vi "Version_4.9_8_on-chip_valves_for25ulSyringe_withModfied_Plunging.vi"() -> ()   [LabVIEW 2020] (continued)
                                n6529 = local write "Initial Plunger Position"(w6934) -> ()
                                }
                                frame #26 {
                                # "Switch to Port-10"
                                # "Port-10 of the pump is conncted to column-2 of chip"
                                n6530 = local read "VISA Refnum in\nfor Pump"() -> (w6937:refnum<visa-resource-name>)
                                n6531 = call "PortChanger (SubVI).vi"("Port Number"="10", "VISA Refnum in"=w6937) -> ()  [unwired: 10 in]
                                }
                                frame #27 {
                                n6532 = local read "Stopper that ends \nthe main loops"() -> (w6938:bool)
                                n6533 = local read "VISA Refnum in\nfor Pump"() -> (w6939:refnum<visa-resource-name>)
                                n6534 = call "ProcessCompletionWaiter (SubVI).vi"("VISA Refnum in"=w6939) -> ()  [unwired: 11 in]
                                n6535 = case shown="True" w6938 {
                                frame False {
                                }
                                frame True {
                                n6536 = local read "VISA Refnum in\nfor Pump"() -> (w6940:refnum<visa-resource-name>)
                                n6537 = call "HardStopCurrentProcess (SubVI).vi"("VISA Refnum in"=w6940) -> ()  [unwired: 11 in]
                                }
                                }
                                }
                                frame #28 {
                                # "Keeps the AMF valve after column-1 open and valve after column-2 closed"
                                n6538 = local read "Buffer-C2 Dispense\nFlow Rate (ul/min)"() -> (w6953:dbl)
                                n6539 = local read "Buffer-C2 Pumping\nResolution"() -> (w6952:T2)
                                n6540 = local read "VISA Refnum in\nfor Pump"() -> (w6955:refnum<visa-resource-name>)
                                n6541 = local write "Pause Data Collection"(FALSE ("Pause Data Collection")) -> ()
                                n6542 = local read "Volume of Syringe"() -> (w6954:dbl)
                                n6543 = call "GoToAbsolutePosition(SubVI).vi"("Absolute Volume Position in Syringe (in ul)"=0.0 ("Volume to be Dispensed"), "Volume of Syringe"=w6954, "Resolution of Pumping"=w6952, "Flow Rate (ul/min)"=w6953, "VISA Refnum in"=w6955) -> ()  [unwired: 6 in, 1 out]
                                n6544 = local read "VISA Refnum in\nfor Valve"() -> (w6949:refnum<visa-resource-name>)
                                n6545 = local read "External Valve \nOPEN"() -> (w6948:string)
                                n6546 = local write "Valve V1 Open"(FALSE ("Valve V1 Open")) -> ()
                                n6547 = local write "Valve V2 Open"(TRUE ("Valve V2 Open")) -> ()
                                n6548 = local write "Valve V3 Open"(TRUE ("Valve V3 Open")) -> ()
                                n6549 = local write "Valve V4 Open"(FALSE ("Valve V4 Open")) -> ()
                                n6550 = call "PortChanger_Valve (SubVI).vi"("Port Number"=w6948, "VISA Refnum in"=w6949) -> ()  [unwired: 10 in]
                                n6551 = local write "Valve V5 Open"(FALSE ("Valve V5 Open")) -> ()
                                n6552 = local write "Valve V6 Open"(FALSE ("Valve V6 Open")) -> ()
                                n6553 = local write "Valve V7 Open"(FALSE ("Valve V7 Open")) -> ()
                                }
                                frame #29 {
                                n6554 = local read "Initial Plunger Position"() -> (w6959:dbl)
                                n6555 = local read "Buffer-C2 Pumping\nResolution"() -> (w6958:T2)
                                n6556 = local read "VISA Refnum in\nfor Pump"() -> (w6960:refnum<visa-resource-name>)
                                n6557 = local read "Volume of Syringe"() -> (w6957:dbl)
                                n6558 = while {
                                tunnel: w6959 -> [w6966]
                                tunnel: w6960 -> [w6965]
                                tunnel: w6958 -> [w6964]
                                tunnel: w6957 -> [w6963]
                                stop <- w6961 stop-if-true
                                n6559 = Wait (ms)(milliseconds to wait=u32 100) -> ()  [unwired: 1 out]
                                n6560 = stacked-sequence {
                                tunnel: w6966 -> [w6972 _]
                                tunnel: w6965 -> [w6971 w6998]
                                tunnel: w6964 -> [w6970 _]
                                tunnel: w6963 -> [w6969 _]
                                tunnel: [_ w6994] -> w6961
                                frame #0 {
                                n6561 = call "AbsolutePlungerPosition (SubVI).vi"("VISA Refnum in"=w6971) -> ("Plunger Position"=w6968:i32)  [unwired: 10 in]
                                n6562 = case shown="\"Standard Pumping\", Default" w6970 {
                                tunnel: w6972 -> [w6977 w6986]
                                tunnel: w6968 -> [w6978 w6985]
                                tunnel: [w6976 w6983] -> w6967
                                tunnel: w6969 -> [w6975 w6984]
                                frame "Standard Pumping", Default {
                                n6563 = Subtract(x=w6977, y=w6978) -> (x-y=w6974:dbl)
                                n6564 = Absolute Value(x=w6974) -> (abs(x)=w6973:dbl)
                                n6565 = Multiply(x=w6973, y=w6975) -> (x*y=w6980:dbl)
                                n6566 = Divide(x=w6980, y=3000.0) -> (x/y=w6976:dbl)
                                }
                                frame "High Resolution Pumping" {
                                n6567 = Subtract(x=w6986, y=w6985) -> (x-y=w6982:dbl)
                                n6568 = Absolute Value(x=w6982) -> (abs(x)=w6981:dbl)
                                n6569 = Multiply(x=w6981, y=w6984) -> (x*y=w6988:dbl)
                                n6570 = Divide(x=w6988, y=24000.0) -> (x/y=w6983:dbl)
                                }
                                }
                                n6571 = local write "Volume being Injected \nin this process"(w6967) -> ()
                                }
                                frame #1 {
                                n6572 = local read "Stopper that ends \nthe main loops"() -> (w6995:bool)
                                n6573 = local read "Divert Buffer-C \ninto Column-2"() -> (w6996:bool)
                                n6574 = local read "Volume being Injected \nin this process"() -> (w6993:dbl)
                                n6575 = call "LSPOneStatus (SubVI).vi"("VISA Refnum in"=w6998) -> ("read buffer"=w7000:string)  [unwired: 10 in]
                                n6576 = call <vilib>:"Trim Whitespace.vi"("string"=w7000) -> ("trimmed string"=w6999:string)  [unwired: 1 in]
                                n6577 = Equal?(x=w6999, y="/0`\u0003") -> (x = y?=w6997:bool)
                                n6578 = Or(x=w6996, y=w6995) -> (x .or. y?=w6991:bool)
                                n6579 = Greater Or Equal?(x=w6993, y=2.0) -> (x >= y?=w6990:bool)
                                n6580 = Or(x=w6991, y=w6990) -> (x .or. y?=w6989:bool)
                                n6581 = Or(x=w6997, y=w6989) -> (x .or. y?=w6994:bool)
                                }
                                }
                                }
                                n6582 = local read "Stopper that ends \nthe main loops"() -> (w6956:bool)
                                n6583 = case shown="True" w6956 {
                                frame False {
                                }
                                frame True {
                                n6584 = local read "VISA Refnum in\nfor Pump"() -> (w7002:refnum<visa-resource-name>)
                                n6585 = call "HardStopCurrentProcess (SubVI).vi"("VISA Refnum in"=w7002) -> ()  [unwired: 11 in]
                                }
                                }
                                }
                                frame #30 {
                                # "Keeps the on-chip valves V4, V5 and V7 open"
                                # "Keeps the AMF valve after column-1 closed and valve after column-2 open"
                                n6586 = local write "Divert Buffer-C \ninto Column-2"(FALSE ("Divert Buffer-C \ninto Column-2")) -> ()
                                n6587 = local read "VISA Refnum in\nfor Pump"() -> (w7007:refnum<visa-resource-name>)
                                n6588 = local read "External Valve \nCLOSED"() -> (w7006:string)
                                n6589 = local write "Valve V3 Open"(FALSE ("Valve V3 Open")) -> ()
                                n6590 = local write "Valve V2 Open"(FALSE ("Valve V2 Open")) -> ()
                                n6591 = local write "Valve V1 Open"(FALSE ("Valve V1 Open")) -> ()
                                n6592 = local write "Valve V4 Open"(TRUE ("Valve V4 Open")) -> ()
                                n6593 = call "PortChanger_Valve (SubVI).vi"("Port Number"=w7006, "VISA Refnum in"=w7007) -> ()  [unwired: 10 in]
                                n6594 = local write "Valve V5 Open"(TRUE ("Valve V5 Open")) -> ()
                                n6595 = local write "Valve V6 Open"(FALSE ("Valve V6 Open")) -> ()
                                n6596 = local write "Valve V7 Open"(TRUE ("Valve V7 Open")) -> ()
                                }
                                frame #31 {
                                n6597 = local read "Initial Plunger Position"() -> (w7016:dbl)
                                n6598 = local read "Buffer-C2 Pumping\nResolution"() -> (w7015:T2)
                                n6599 = local read "VISA Refnum in\nfor Pump"() -> (w7017:refnum<visa-resource-name>)
                                n6600 = local read "Volume of Syringe"() -> (w7014:dbl)
                                n6601 = while {
                                tunnel: w7016 -> [w7023]
                                tunnel: w7017 -> [w7022]
                                tunnel: w7015 -> [w7021]
                                tunnel: w7014 -> [w7020]
                                stop <- w7018 stop-if-true
                                n6602 = Wait (ms)(milliseconds to wait=u32 100) -> ()  [unwired: 1 out]
                                n6603 = stacked-sequence {
                                tunnel: w7023 -> [w7029 _]
                                tunnel: w7022 -> [w7028 w7051]
                                tunnel: w7021 -> [w7027 _]
                                tunnel: w7020 -> [w7026 _]
                                tunnel: [_ w7049] -> w7018
                                frame #0 {
                                n6604 = call "AbsolutePlungerPosition (SubVI).vi"("VISA Refnum in"=w7028) -> ("Plunger Position"=w7025:i32)  [unwired: 10 in]
                                n6605 = case shown="\"Standard Pumping\", Default" w7027 {
                                tunnel: w7029 -> [w7034 w7043]
                                tunnel: w7025 -> [w7035 w7042]
                                tunnel: [w7033 w7040] -> w7024
                                tunnel: w7026 -> [w7032 w7041]
                                frame "Standard Pumping", Default {
                                n6606 = Subtract(x=w7034, y=w7035) -> (x-y=w7031:dbl)
                                n6607 = Absolute Value(x=w7031) -> (abs(x)=w7030:dbl)
                                n6608 = Multiply(x=w7030, y=w7032) -> (x*y=w7037:dbl)
                                n6609 = Divide(x=w7037, y=3000.0) -> (x/y=w7033:dbl)
                                }
                                frame "High Resolution Pumping" {
                                n6610 = Subtract(x=w7043, y=w7042) -> (x-y=w7039:dbl)
                                n6611 = Absolute Value(x=w7039) -> (abs(x)=w7038:dbl)
                                n6612 = Multiply(x=w7038, y=w7041) -> (x*y=w7045:dbl)
                                n6613 = Divide(x=w7045, y=24000.0) -> (x/y=w7040:dbl)
                                }
                                }
                                n6614 = local write "Volume being Injected \nin this process"(w7024) -> ()
                                }
                                frame #1 {
                                n6615 = call "LSPOneStatus (SubVI).vi"("VISA Refnum in"=w7051) -> ("read buffer"=w7053:string)  [unwired: 10 in]
                                n6616 = call <vilib>:"Trim Whitespace.vi"("string"=w7053) -> ("trimmed string"=w7052:string)  [unwired: 1 in]
                                n6617 = Equal?(x=w7052, y="/0`\u0003") -> (x = y?=w7050:bool)
                                n6618 = local read "Stopper that ends \nthe main loops"() -> (w7047:bool)
                                n6619 = local read "Divert Sample \nonto Grid"() -> (w7048:bool)
                                n6620 = Or(x=w7048, y=w7047) -> (x .or. y?=w7046:bool)
                                n6621 = Or(x=w7050, y=w7046) -> (x .or. y?=w7049:bool)
                                }
                                }
                                }
                                n6622 = local read "Stopper that ends \nthe main loops"() -> (w7013:bool)
                                n6623 = case shown="True" w7013 {
                                frame False {
                                }
                                frame True {
                                n6624 = local read "VISA Refnum in\nfor Pump"() -> (w7055:refnum<visa-resource-name>)
                                n6625 = call "HardStopCurrentProcess (SubVI).vi"("VISA Refnum in"=w7055) -> ()  [unwired: 11 in]
                                }
                                }
                                }
                                frame #32 {
                                n6626 = local read "Volume being Injected \nin this process"() -> (w7058:dbl)
                                n6627 = local read "VISA Refnum in\nfor Pump"() -> (w7060:refnum<visa-resource-name>)
                                n6628 = call "AbsolutePlungerPosition (SubVI).vi"("VISA Refnum in"=w7060) -> ("Plunger Position"=w7059:i32)  [unwired: 10 in]
                                n6629 = local write "Pause Data Collection"(TRUE) -> ()
                                n6630 = local write "True Volume being \ninjected in this\nprocess"(w7058) -> ()
                                n6631 = local write "Position\nNow"(w7059) -> ()
                                n6632 = Wait (ms)(milliseconds to wait=u32 500) -> ()  [unwired: 1 out]
                                }
                                frame #33 {
                                # "Sample Deposition onto EM-Grid"
                                n6633 = local read "Divert Sample \nonto Grid"() -> (w7061:bool)
                                n6634 = case shown="True" w7061 {
                                frame False {
                                }
                                frame True {
                                n6635 = stacked-sequence {
                                frame #0 {
                                # "Discard the initial volume of fluid that is present in the channel prior to detection"
                                n6636 = local read "Buffer-C2 Pumping\nResolution"() -> (w7072:T2)
                                n6637 = local read "Initial Plunger Position"() -> (w7071:dbl)
                                n6638 = local read "VISA Refnum in\nfor Pump"() -> (w7073:refnum<visa-resource-name>)
                                n6639 = local read "Position\nNow"() -> (w7069:dbl)
                                n6640 = local read "Volume of Syringe"() -> (w7070:dbl)
                                n6641 = local write "Pause Data Collection"(FALSE) -> ()
                                n6642 = while {
                                tunnel: w7073 -> [w7083]
                                tunnel: w7072 -> [w7082]
                                tunnel: w7071 -> [w7078]
                                tunnel: w7070 -> [w7081]
                                tunnel: w7069 -> [w7077]
                                stop <- w7079 stop-if-true
                                n6643 = stacked-sequence {
                                tunnel: w7083 -> [w7089 w7111 w7143]
                                tunnel: w7082 -> [w7088 w7110 _]
                                tunnel: w7078 -> [w7086 _ _]
                                tunnel: w7081 -> [w7085 w7108 _]
                                tunnel: [_ _ w7137] -> w7079
                                tunnel: w7077 -> [_ w7106 _]
                                frame #0 {
                                # "From here on 'True Volume being injected \nin this process' represents the true total \nvolume in this process"
                                n6644 = call "AbsolutePlungerPosition (SubVI).vi"("VISA Refnum in"=w7089) -> ("Plunger Position"=w7087:i32)  [unwired: 10 in]
                                n6645 = case shown="..\"Standard Pumping\"" w7088 {
                                tunnel: w7087 -> [w7097 w7105]
                                tunnel: w7086 -> [w7096 w7104]
                                tunnel: w7085 -> [w7093 w7101]
                                tunnel: [w7090 w7098] -> w7084
                                frame .."Standard Pumping" {
                                n6646 = Subtract(x=w7097, y=w7096) -> (x-y=w7095:dbl)
                                n6647 = Absolute Value(x=w7095) -> (abs(x)=w7094:dbl)
                                n6648 = Multiply(x=w7094, y=w7093) -> (x*y=w7092:dbl)
                                n6649 = Divide(x=w7092, y=3000.0) -> (x/y=w7090:dbl)
                                }
                                frame "High Resolution Pumping".. {
                                n6650 = Subtract(x=w7105, y=w7104) -> (x-y=w7103:dbl)
                                n6651 = Absolute Value(x=w7103) -> (abs(x)=w7102:dbl)
                                n6652 = Multiply(x=w7102, y=w7101) -> (x*y=w7100:dbl)
                                n6653 = Divide(x=w7100, y=24000.0) -> (x/y=w7098:dbl)
                                }
                                }
                                n6654 = local write "True Volume being \ninjected in this\nprocess"(w7084) -> ()
                                }
                                frame #1 {
                                # "From here on 'Volume being injected \nin this process' represents the volume \nin this sub process"
                                n6655 = call "AbsolutePlungerPosition (SubVI).vi"("VISA Refnum in"=w7111) -> ("Plunger Position"=w7109:i32)  [unwired: 10 in]
                                n6656 = case shown="..\"Standard Pumping\"" w7110 {
                                tunnel: w7109 -> [w7119 w7127]
                                tunnel: w7106 -> [w7118 w7126]
                                tunnel: w7108 -> [w7115 w7123]
                                tunnel: [w7112 w7120] -> w7107
                                frame .."Standard Pumping" {
                                n6657 = Subtract(x=w7119, y=w7118) -> (x-y=w7117:dbl)
                                n6658 = Absolute Value(x=w7117) -> (abs(x)=w7116:dbl)
                                n6659 = Multiply(x=w7116, y=w7115) -> (x*y=w7114:dbl)
                                n6660 = Divide(x=w7114, y=3000.0) -> (x/y=w7112:dbl)
                                }
                                frame "High Resolution Pumping".. {
                                n6661 = Subtract(x=w7127, y=w7126) -> (x-y=w7125:dbl)
                                n6662 = Absolute Value(x=w7125) -> (abs(x)=w7124:dbl)
                                n6663 = Multiply(x=w7124, y=w7123) -> (x*y=w7122:dbl)
                                n6664 = Divide(x=w7122, y=24000.0) -> (x/y=w7120:dbl)
                                }
                                }
                                n6665 = local write "Volume being Injected \nin this process"(w7107) -> ()
                                }
                                frame #2 {
                                n6666 = local read "Discard Volume"() -> (w7131:dbl)
                                n6667 = local read "Discard fluid \nprior to 1st \ndeposition"() -> (w7136:bool)
                                n6668 = local read "Volume being Injected \nin this process"() -> (w7135:dbl)
                                n6669 = Greater Or Equal?(x=w7135, y=w7131) -> (x >= y?=w7133:bool)
                                n6670 = call "AbsolutePlungerPositionStatus (SubVI).vi"("VISA Refnum in"=w7143) -> ("read buffer"=w7142:string)  [unwired: 10 in]
                                n6671 = local read "Stop for End of \nExperiment \nand Data Writing"() -> (w7129:bool)
                                n6672 = call <vilib>:"Trim Whitespace.vi"("string"=w7142) -> ("trimmed string"=w7141:string)  [unwired: 1 in]
                                n6673 = Not(x=w7136) -> (.not. x?=w7134:bool)
                                n6674 = Equal?(x=w7141, y="/0`\u0003") -> (x = y?=w7139:bool)
                                n6675 = Or(x=w7134, y=w7133) -> (x .or. y?=w7132:bool)
                                n6676 = local read "Re-SEC"() -> (w7130:bool)
                                n6677 = Or(x=w7129, y=w7130) -> (x .or. y?=w7128:bool)
                                n6678 = Or(x=w7132, y=w7128) -> (x .or. y?=w7138:bool)
                                n6679 = Or(x=w7139, y=w7138) -> (x .or. y?=w7137:bool)
                                }
                                }
                                n6680 = Wait (ms)(milliseconds to wait=u32 100) -> ()  [unwired: 1 out]
                                }
                                n6681 = local write "Valve V4 Open"(TRUE ("Valve V4 Open")) -> ()
                                n6682 = local write "Valve V3 Open"(FALSE ("Valve V3 Open")) -> ()
                                n6683 = local write "Valve V2 Open"(FALSE ("Valve V2 Open")) -> ()
                                n6684 = local write "Valve V1 Open"(FALSE ("Valve V1 Open")) -> ()
                                n6685 = local write "Valve V5 Open"(TRUE ("Valve V5 Open")) -> ()
                                n6686 = local write "Valve V6 Open"(TRUE ("Valve V6 Open")) -> ()
                                n6687 = local write "Valve V7 Open"(FALSE ("Valve V7 Open")) -> ()
                                n6688 = local write "Volume being Injected \nin this process"(0.0) -> ()
                                }
                                frame #1 {
                                # "Keeps the on-chip valve V1, V2 and V3 closed,\nHalts also deposition onto the grid\nand waits for the 1st redeposit command. Once the command is issued\nit starts pumpoing and moves onto the next frame"
                                n6689 = stacked-sequence {
                                frame #0 {
                                n6690 = local write "Valve V5 Open"(FALSE ("Valve V5 Open")) -> ()
                                n6691 = local write "Valve V1 Open"(FALSE ("Valve V1 Open")) -> ()
                                n6692 = local read "VISA Refnum in\nfor Pump"() -> (w7153:refnum<visa-resource-name>)
                                n6693 = local write "Valve V2 Open"(FALSE ("Valve V2 Open")) -> ()
                                n6694 = local write "Valve V6 Open"(FALSE ("Valve V6 Open")) -> ()
                                n6695 = local write "Re-deposit Sample\nonto Grid"(FALSE ("Redeposit Sample\nonto Grid")) -> ()
                                n6696 = local write "Pause Data Collection"(TRUE ("Pause Data Collection")) -> ()
                                n6697 = call "HardStopCurrentProcess (SubVI).vi"("VISA Refnum in"=w7153) -> ()  [unwired: 11 in]
                                n6698 = local write "Valve V7 Open"(FALSE ("Valve V7 Open")) -> ()
                                n6699 = local write "Valve V3 Open"(FALSE ("Valve V3 Open")) -> ()
                                n6700 = local write "Valve V4 Open"(FALSE ("Valve V4 Open")) -> ()
                                }
                                frame #1 {
                                n6701 = while {
                                stop <- w7159 stop-if-true
                                n6702 = local read "Stop for End of \nExperiment \nand Data Writing"() -> (w7157:bool)
                                n6703 = local read "Re-deposit Sample\nonto Grid"() -> (w7160:bool)
                                n6704 = local read "Re-SEC"() -> (w7158:bool)
                                n6705 = Or(x=w7157, y=w7158) -> (x .or. y?=w7156:bool)
                                n6706 = Or(x=w7160, y=w7156) -> (x .or. y?=w7159:bool)
                                }
                                n6707 = local write "Discard fluid \nprior to 1st \ndeposition"(FALSE ("Discard fluid \nprior to 1st \ndeposition")) -> ()
                                n6708 = One Button Dialog(message="Do you want to deposit sample on another grid? If yes, turn on 'Re-deposit Sample onto Grid'. Else turn on Re-SEC to do SEC again or STOP to end the experiment") -> ()  [unwired: 1 in, 1 out]
                                }
                                frame #2 {
                                n6709 = local write "Valve V6 Open"(TRUE ("Valve V3 Open")) -> ()
                                n6710 = local write "Valve V4 Open"(TRUE ("Valve V1 Open")) -> ()
                                n6711 = local write "Valve V5 Open"(TRUE ("Valve V2 Open")) -> ()
                                n6712 = local write "Valve V7 Open"(FALSE ("Valve V7 Open")) -> ()
                                }
                                frame #3 {
                                n6713 = local read "Re-deposit Sample\nonto Grid"() -> (w7165:bool)
                                n6714 = case shown="True" w7165 {
                                frame False {
                                n6715 = local write "Suction On/Off"(FALSE ("Suction On/Off")) -> ()
                                }
                                frame True {
                                n6716 = stacked-sequence {
                                frame #0 {
                                n6717 = local read "VISA Refnum in\nfor Pump"() -> (w7168:refnum<visa-resource-name>)
                                n6718 = call "AbsolutePlungerPosition (SubVI).vi"("VISA Refnum in"=w7168) -> ("Plunger Position"=w7167:i32)  [unwired: 10 in]
                                n6719 = local write "Position\nNow"(w7167) -> ()
                                }
                                frame #1 {
                                n6720 = local read "Buffer-C2 Pumping\nResolution"() -> (w7170:T2)
                                n6721 = case shown="\"Standard Pumping\", Default" w7170 {
                                tunnel: [w7171 w7182] -> w7169
                                frame "Standard Pumping", Default {
                                n6722 = local read "Buffer-C2 Volume \nto be Pumped"() -> (w7174:dbl)
                                n6723 = local read "Volume of Syringe"() -> (w7177:dbl)
                                n6724 = local read "Initial Plunger Position"() -> (w7181:dbl)
                                n6725 = local read "Position\nNow"() -> (w7180:dbl)
                                n6726 = Subtract(x=w7181, y=w7180) -> (x-y=w7179:dbl)
                                n6727 = Absolute Value(x=w7179) -> (abs(x)=w7178:dbl)
                                n6728 = Multiply(x=w7178, y=w7177) -> (x*y=w7176:dbl)
                                n6729 = Divide(x=w7176, y=3000.0) -> (x/y=w7173:dbl)
                                n6730 = Subtract(x=w7173, y=w7174) -> (x-y=w7172:dbl)
                                n6731 = Absolute Value(x=w7172) -> (abs(x)=w7171:dbl)
                                }
                                frame "High Resolution Pumping" {
                                n6732 = local read "Buffer-C2 Volume \nto be Pumped"() -> (w7185:dbl)
                                n6733 = local read "Volume of Syringe"() -> (w7188:dbl)
                                n6734 = local read "Initial Plunger Position"() -> (w7192:dbl)
                                n6735 = local read "Position\nNow"() -> (w7191:dbl)
                                n6736 = Subtract(x=w7192, y=w7191) -> (x-y=w7190:dbl)
                                n6737 = Absolute Value(x=w7190) -> (abs(x)=w7189:dbl)
                                n6738 = Multiply(x=w7189, y=w7188) -> (x*y=w7187:dbl)
                                n6739 = Divide(x=w7187, y=24000.0) -> (x/y=w7184:dbl)
                                n6740 = Subtract(x=w7184, y=w7185) -> (x-y=w7183:dbl)
                                n6741 = Absolute Value(x=w7183) -> (abs(x)=w7182:dbl)
                                }
                                }
                                n6742 = local write "Buffer-C Volume\nleft to be Pumped"(w7169) -> ()
                                }
                                frame #2 {
                                n6743 = local read "Buffer-C2 Dispense\nFlow Rate (ul/min)"() -> (w7196:dbl)
                                n6744 = local read "Buffer-C2 Pumping\nResolution"() -> (w7195:T2)
                                n6745 = local read "VISA Refnum in\nfor Pump"() -> (w7198:refnum<visa-resource-name>)
                                n6746 = local read "Volume of Syringe"() -> (w7197:dbl)
                                n6747 = call "GoToAbsolutePosition(SubVI).vi"("Absolute Volume Position in Syringe (in ul)"=0.0, "Volume of Syringe"=w7197, "Resolution of Pumping"=w7195, "Flow Rate (ul/min)"=w7196, "VISA Refnum in"=w7198) -> ()  [unwired: 6 in, 1 out]
                                n6748 = local write "Suction On/Off"(FALSE ("Suction On/Off")) -> ()
                                }
                                }
                                }
                                }
                                }
                                frame #4 {
                                n6749 = local read "Stop for End of \nExperiment \nand Data Writing"() -> (w7200:bool)
                                n6750 = local read "Re-SEC"() -> (w7201:bool)
                                n6751 = Or(x=w7200, y=w7201) -> (x .or. y?=w7199:bool)
                                n6752 = case shown="True" w7199 {
                                frame False {
                                }
                                frame True {
                                n6753 = local read "VISA Refnum in\nfor Pump"() -> (w7202:refnum<visa-resource-name>)
                                n6754 = call "HardStopCurrentProcess (SubVI).vi"("VISA Refnum in"=w7202) -> ()  [unwired: 11 in]
                                }
                                }
                                }
                                }
                                }
                                frame #2 {
                                # "Keeps the on-chip valve V1, V2 Open and V3 closed"
                                n6755 = while {
                                stop <- w7208 stop-if-true
                                n6756 = local read "Suction On/Off"() -> (w7209:bool)
                                n6757 = case shown="True" w7209 {
                                frame False {
                                n6758 = local read "Buffer-C2 Pumping\nResolution"() -> (w7215:T2)
                                n6759 = local read "Initial Plunger Position"() -> (w7214:dbl)
                                n6760 = local read "VISA Refnum in\nfor Pump"() -> (w7216:refnum<visa-resource-name>)
                                n6761 = local read "Position\nNow"() -> (w7212:dbl)
                                n6762 = local read "Volume of Syringe"() -> (w7213:dbl)
                                n6763 = local write "Volume being Injected \nin this process"(0.0) -> ()
                                n6764 = local write "Pause Data Collection"(FALSE) -> ()
                                n6765 = while {
                                tunnel: w7216 -> [w7223]
                                tunnel: w7215 -> [w7222]
                                tunnel: w7214 -> [w7218]
                                tunnel: w7213 -> [w7221]
                                tunnel: w7212 -> [w7217]
                                stop <- w7219 stop-if-true
                                n6766 = stacked-sequence {
                                tunnel: w7223 -> [w7229 w7251 w7276]
                                tunnel: w7222 -> [w7228 w7250 _]
                                tunnel: w7218 -> [w7226 _ _]
                                tunnel: w7221 -> [w7225 w7248 _]
                                tunnel: [_ _ w7268] -> w7219
                                tunnel: w7217 -> [_ w7246 _]
                                frame #0 {
                                # "From here on 'True Volume being injected \nin this process' represents the true total \nvolume in this process"
                                n6767 = call "AbsolutePlungerPosition (SubVI).vi"("VISA Refnum in"=w7229) -> ("Plunger Position"=w7227:i32)  [unwired: 10 in]
                                n6768 = case shown="..\"Standard Pumping\"" w7228 {
                                tunnel: w7227 -> [w7237 w7245]
                                tunnel: w7226 -> [w7236 w7244]
                                tunnel: w7225 -> [w7233 w7241]
                                tunnel: [w7230 w7238] -> w7224
                                frame .."Standard Pumping" {
                                n6769 = Subtract(x=w7237, y=w7236) -> (x-y=w7235:dbl)
                                n6770 = Absolute Value(x=w7235) -> (abs(x)=w7234:dbl)
                                n6771 = Multiply(x=w7234, y=w7233) -> (x*y=w7232:dbl)
                                n6772 = Divide(x=w7232, y=3000.0) -> (x/y=w7230:dbl)
                                }
                                frame "High Resolution Pumping".. {
                                n6773 = Subtract(x=w7245, y=w7244) -> (x-y=w7243:dbl)
                                n6774 = Absolute Value(x=w7243) -> (abs(x)=w7242:dbl)
                                n6775 = Multiply(x=w7242, y=w7241) -> (x*y=w7240:dbl)
                                n6776 = Divide(x=w7240, y=24000.0) -> (x/y=w7238:dbl)
                                }
                                }
                                n6777 = local write "True Volume being \ninjected in this\nprocess"(w7224) -> ()
                                }
                                frame #1 {
                                # "From here on 'Volume being injected \nin this process' represents the volume \nin this sub process"
                                n6778 = call "AbsolutePlungerPosition (SubVI).vi"("VISA Refnum in"=w7251) -> ("Plunger Position"=w7249:i32)  [unwired: 10 in]
                                n6779 = case shown="..\"Standard Pumping\"" w7250 {
                                tunnel: w7249 -> [w7259 w7267]
                                tunnel: w7246 -> [w7258 w7266]
                                tunnel: w7248 -> [w7255 w7263]
                                tunnel: [w7252 w7260] -> w7247
                                frame .."Standard Pumping" {
                                n6780 = Subtract(x=w7259, y=w7258) -> (x-y=w7257:dbl)
                                n6781 = Absolute Value(x=w7257) -> (abs(x)=w7256:dbl)
                                n6782 = Multiply(x=w7256, y=w7255) -> (x*y=w7254:dbl)
                                n6783 = Divide(x=w7254, y=3000.0) -> (x/y=w7252:dbl)
                                }
                                frame "High Resolution Pumping".. {
                                n6784 = Subtract(x=w7267, y=w7266) -> (x-y=w7265:dbl)
                                n6785 = Absolute Value(x=w7265) -> (abs(x)=w7264:dbl)
                                n6786 = Multiply(x=w7264, y=w7263) -> (x*y=w7262:dbl)
                                n6787 = Divide(x=w7262, y=24000.0) -> (x/y=w7260:dbl)
                                }
                                }
                                n6788 = local write "Volume being Injected \nin this process"(w7247) -> ()
                                }
                                frame #2 {
                                n6789 = local read "Stop for End of \nExperiment \nand Data Writing"() -> (w7271:bool)
                                n6790 = local read "Suction On/Off"() -> (w7272:bool)
                                n6791 = call "AbsolutePlungerPositionStatus (SubVI).vi"("VISA Refnum in"=w7276) -> ("read buffer"=w7275:string)  [unwired: 10 in]
                                n6792 = call <vilib>:"Trim Whitespace.vi"("string"=w7275) -> ("trimmed string"=w7274:string)  [unwired: 1 in]
                                n6793 = Equal?(x=w7274, y="/0`\u0003") -> (x = y?=w7270:bool)
                                n6794 = Or(x=w7272, y=w7271) -> (x .or. y?=w7269:bool)
                                n6795 = Or(x=w7270, y=w7269) -> (x .or. y?=w7268:bool)
                                }
                                }
                                n6796 = Wait (ms)(milliseconds to wait=u32 100) -> ()  [unwired: 1 out]
                                }
                                }
                                frame True {
                                n6797 = stacked-sequence {
                                frame #0 {
                                n6798 = local read "Suction Pressure\nfor EM-grid \nDeposition (mbar)"() -> (w7281:sgl)
                                n6799 = local write "Valve V4 Open"(FALSE ("Valve V4 Open")) -> ()
                                n6800 = local read "VISA Refnum in\nfor Pump"() -> (w7284:refnum<visa-resource-name>)
                                n6801 = local write "Valve V5 Open"(FALSE ("Valve V1 Open")) -> ()
                                n6802 = local write "Suction pressure \nfor grid deposition"(w7281) -> ()
                                n6803 = local write "Re-deposit Sample\nonto Grid"(FALSE ("Redeposit Sample\nonto Grid")) -> ()
                                n6804 = local write "Pause Data Collection"(TRUE ("Pause Data Collection")) -> ()
                                n6805 = call "HardStopCurrentProcess (SubVI).vi"("VISA Refnum in"=w7284) -> ()  [unwired: 11 in]
                                n6806 = local write "Valve V6 Open"(TRUE ("Valve V2 Open")) -> ()
                                n6807 = local write "Valve V7 Open"(TRUE ("Valve V3 Open")) -> ()
                                }
                                frame #1 {
                                n6808 = call <vilib>:"fgt init.vi"() -> ("error out"=w7285:errorcluster)  [unwired: 11 in]
                                n6809 = while {
                                tunnel: [w7288] -> w7286
                                tunnel: w7285 -> [w7287]
                                stop <- w7291 stop-if-true
                                # "'5' corresponds to 2nd positin in the line-up series"
                                n6810 = local read "Stop for End of \nExperiment \nand Data Writing"() -> (w7292:bool)
                                n6811 = local read "Suction Pressure\nfor EM-grid \nDeposition (mbar)"() -> (w7289:sgl)
                                n6812 = call <vilib>:"fgt set pressure.vi"("error in (no error)"=w7287, "pressure"=w7289, "pressureIndex"=u32 1) -> ("error out"=w7288:errorcluster)  [unwired: 8 in]
                                n6813 = local read "Suction On/Off"() -> (w7294:bool)
                                n6814 = Not(x=w7294) -> (.not. x?=w7293:bool)
                                n6815 = Wait (ms)(milliseconds to wait=u32 10) -> ()  [unwired: 1 out]
                                n6816 = Or(x=w7293, y=w7292) -> (x .or. y?=w7291:bool)
                                }
                                n6817 = call <vilib>:"fgt close.vi"("error in (no error)"=w7286) -> ()  [unwired: 10 in, 1 out]
                                }
                                frame #2 {
                                n6818 = call <vilib>:"fgt init.vi"() -> ("error out"=w7297:errorcluster)  [unwired: 11 in]
                                n6819 = while {
                                tunnel: w7297 -> [w7300]
                                tunnel: [w7298] -> w7296
                                stop <- w7306 stop-if-true
                                n6820 = local read "Stop for End of \nExperiment \nand Data Writing"() -> (w7302:bool)
                                n6821 = local read "Suction On/Off"() -> (w7304:bool)
                                n6822 = call <vilib>:"fgt set pressure.vi"("error in (no error)"=w7300, "pressure"=sgl 0.0, "pressureIndex"=u32 1) -> ("error out"=w7298:errorcluster)  [unwired: 8 in]
                                n6823 = Not(x=w7304) -> (.not. x?=w7303:bool)
                                n6824 = Wait (ms)(milliseconds to wait=u32 10) -> ()  [unwired: 1 out]
                                n6825 = Or(x=w7303, y=w7302) -> (x .or. y?=w7306:bool)
                                }
                                n6826 = call <vilib>:"fgt close.vi"("error in (no error)"=w7296) -> ()  [unwired: 10 in, 1 out]
                                }
                                frame #3 {
                                n6827 = local write "Valve V7 Open"(FALSE ("Valve V3 Open")) -> ()
                                n6828 = local write "Valve V5 Open"(FALSE ("Valve V1 Open")) -> ()
                                n6829 = local write "Valve V6 Open"(FALSE ("Valve V2 Open")) -> ()
                                n6830 = local write "Valve V4 Open"(FALSE ("Valve V4 Open")) -> ()
                                }
                                frame #4 {
                                n6831 = while {
                                stop <- w7315 stop-if-true
                                n6832 = local read "Stop for End of \nExperiment \nand Data Writing"() -> (w7313:bool)
                                n6833 = local read "Re-deposit Sample\nonto Grid"() -> (w7316:bool)
                                n6834 = local read "Re-SEC"() -> (w7314:bool)
                                n6835 = Or(x=w7313, y=w7314) -> (x .or. y?=w7312:bool)
                                n6836 = Or(x=w7316, y=w7312) -> (x .or. y?=w7315:bool)
                                }
                                n6837 = One Button Dialog(message="Do you want to deposit sample on another grid? If yes, turn on 'Re-deposit Sample onto Grid'. Else turn on Re-SEC to do SEC again or STOP to end the experiment") -> ()  [unwired: 1 in, 1 out]
                                }
                                frame #5 {
                                n6838 = local write "Valve V4 Open"(TRUE ("Valve V4 Open")) -> ()
                                n6839 = local write "Valve V7 Open"(FALSE ("Valve V3 Open")) -> ()
                                n6840 = local write "Valve V5 Open"(TRUE ("Valve V1 Open")) -> ()
                                n6841 = local write "Valve V6 Open"(TRUE ("Valve V2 Open")) -> ()
                                }
                                frame #6 {
                                n6842 = local read "Re-deposit Sample\nonto Grid"() -> (w7321:bool)
                                n6843 = case shown="True" w7321 {
                                frame False {
                                n6844 = local write "Suction On/Off"(FALSE ("Suction On/Off")) -> ()
                                }
                                frame True {
                                n6845 = stacked-sequence {
                                frame #0 {
                                n6846 = local read "VISA Refnum in\nfor Pump"() -> (w7324:refnum<visa-resource-name>)
                                n6847 = call "AbsolutePlungerPosition (SubVI).vi"("VISA Refnum in"=w7324) -> ("Plunger Position"=w7323:i32)  [unwired: 10 in]
                                n6848 = local write "Position\nNow"(w7323) -> ()
                                }
                                frame #1 {
                                n6849 = local read "Buffer-C2 Pumping\nResolution"() -> (w7326:T2)
                                n6850 = case shown="\"Standard Pumping\", Default" w7326 {
                                tunnel: [w7327 w7338] -> w7325
                                frame "Standard Pumping", Default {
                                n6851 = local read "Buffer-C2 Volume \nto be Pumped"() -> (w7330:dbl)
                                n6852 = local read "Volume of Syringe"() -> (w7333:dbl)
                                n6853 = local read "Initial Plunger Position"() -> (w7337:dbl)
                                n6854 = local read "Position\nNow"() -> (w7336:dbl)
                                n6855 = Subtract(x=w7337, y=w7336) -> (x-y=w7335:dbl)
                                n6856 = Absolute Value(x=w7335) -> (abs(x)=w7334:dbl)
                                n6857 = Multiply(x=w7334, y=w7333) -> (x*y=w7332:dbl)
                                n6858 = Divide(x=w7332, y=3000.0) -> (x/y=w7329:dbl)
                                n6859 = Subtract(x=w7329, y=w7330) -> (x-y=w7328:dbl)
                                n6860 = Absolute Value(x=w7328) -> (abs(x)=w7327:dbl)
                                }
                                frame "High Resolution Pumping" {
                                n6861 = local read "Buffer-C2 Volume \nto be Pumped"() -> (w7341:dbl)
                                n6862 = local read "Volume of Syringe"() -> (w7344:dbl)
                                n6863 = local read "Initial Plunger Position"() -> (w7348:dbl)
                                n6864 = local read "Position\nNow"() -> (w7347:dbl)
                                n6865 = Subtract(x=w7348, y=w7347) -> (x-y=w7346:dbl)
                                n6866 = Absolute Value(x=w7346) -> (abs(x)=w7345:dbl)
                                n6867 = Multiply(x=w7345, y=w7344) -> (x*y=w7343:dbl)
                                n6868 = Divide(x=w7343, y=24000.0) -> (x/y=w7340:dbl)
                                n6869 = Subtract(x=w7340, y=w7341) -> (x-y=w7339:dbl)
                                n6870 = Absolute Value(x=w7339) -> (abs(x)=w7338:dbl)
                                }
                                }
                                n6871 = local write "Buffer-C Volume\nleft to be Pumped"(w7325) -> ()
                                }
                                frame #2 {
                                n6872 = local read "Buffer-C2 Dispense\nFlow Rate (ul/min)"() -> (w7352:dbl)
                                n6873 = local read "Buffer-C2 Pumping\nResolution"() -> (w7351:T2)
                                n6874 = local read "VISA Refnum in\nfor Pump"() -> (w7354:refnum<visa-resource-name>)
                                n6875 = local read "Volume of Syringe"() -> (w7353:dbl)
                                n6876 = call "GoToAbsolutePosition(SubVI).vi"("Absolute Volume Position in Syringe (in ul)"=0.0, "Volume of Syringe"=w7353, "Resolution of Pumping"=w7351, "Flow Rate (ul/min)"=w7352, "VISA Refnum in"=w7354) -> ()  [unwired: 6 in, 1 out]
                                n6877 = local write "Suction On/Off"(FALSE ("Suction On/Off")) -> ()
                                }
                                }
                                }
                                }
                                }
                                frame #7 {
                                n6878 = local read "Stop for End of \nExperiment \nand Data Writing"() -> (w7357:bool)
                                n6879 = local read "Re-SEC"() -> (w7356:bool)
                                n6880 = Or(x=w7357, y=w7356) -> (x .or. y?=w7355:bool)
                                n6881 = case shown="True" w7355 {
                                frame False {
                                }
                                frame True {
                                n6882 = local read "VISA Refnum in\nfor Pump"() -> (w7358:refnum<visa-resource-name>)
                                n6883 = call "HardStopCurrentProcess (SubVI).vi"("VISA Refnum in"=w7358) -> ()  [unwired: 11 in]
                                }
                                }
                                }
                                }
                                }
                                }
                                n6884 = local read "Stop for End of \nExperiment \nand Data Writing"() -> (w7204:bool)
                                n6885 = local read "Divert Sample \nonto Grid"() -> (w7207:bool)
                                n6886 = local read "Re-SEC"() -> (w7205:bool)
                                n6887 = Not(x=w7207) -> (.not. x?=w7206:bool)
                                n6888 = Or(x=w7204, y=w7205) -> (x .or. y?=w7203:bool)
                                n6889 = Or(x=w7206, y=w7203) -> (x .or. y?=w7208:bool)
                                }
                                }
                                }
                                n6890 = local write "Discard fluid \nprior to 1st \ndeposition"(TRUE ("Discard fluid \nprior to 1st \ndeposition")) -> ()
                                }
                                }
                                }
                                frame #34 {
                                n6891 = local read "VISA Refnum in\nfor Valve"() -> (w7360:refnum<visa-resource-name>)
                                n6892 = local read "External Valve \nOPEN"() -> (w7359:string)
                                n6893 = Wait (ms)(milliseconds to wait=u32 500) -> ()  [unwired: 1 out]
                                n6894 = call "PortChanger_Valve (SubVI).vi"("Port Number"=w7359, "VISA Refnum in"=w7360) -> ()  [unwired: 10 in]
                                }
                                frame #35 {
                                n6895 = local read "Stopper that ends \nthe main loops"() -> (w7363:bool)
                                n6896 = Wait (ms)(milliseconds to wait=u32 500) -> ()  [unwired: 1 out]
                                n6897 = case shown="True" w7363 {
                                frame False {
                                }
                                frame True {
                                n6898 = local read "VISA Refnum in\nfor Pump"() -> (w7367:refnum<visa-resource-name>)
                                n6899 = call "HardStopCurrentProcess (SubVI).vi"("VISA Refnum in"=w7367) -> ()  [unwired: 11 in]
                                }
                                }
                                n6900 = local write "Pause Data Collection"(TRUE ("Pause Data Collection")) -> ()
                                n6901 = local write "Start the Process"(FALSE ("Start the Process")) -> ()
                                n6902 = local write "Divert Sample \nonto Grid"(FALSE ("Divert Sample \nonto Grid")) -> ()
                                }
                                frame #36 {
                                n6903 = local read "Stop for End of \nExperiment \nand Data Writing"() -> (w7374:bool)
                                n6904 = local read "Start the Process"() -> (w7373:bool)
                                n6905 = Or(x=w7373, y=w7374) -> (x .or. y?=w7372:bool)
                                n6906 = case shown="True" w7372 {
                                frame False {
                                n6907 = while {
                                stop <- w7380 stop-if-true
                                n6908 = local read "Stop for End of \nExperiment \nand Data Writing"() -> (w7382:bool)
                                n6909 = local read "Start the Process"() -> (w7381:bool)
                                n6910 = Or(x=w7381, y=w7382) -> (x .or. y?=w7380:bool)
                                n6911 = Wait (ms)(milliseconds to wait=u32 100) -> ()  [unwired: 1 out]
                                }
                                n6912 = One Button Dialog(message="Do you want to re-introduce sample into column-2 and elute? If yes, adjust the re-introduction volume into column-2 and elution parameters for column-2 and turn on the 'Start the Process' button . If no, turn on the 'Stop for End of Experiment and Data Writing'.") -> ()  [unwired: 1 in, 1 out]
                                }
                                frame True {
                                n6913 = local read "Stop for End of \nExperiment \nand Data Writing"() -> (w7383:bool)
                                n6914 = case shown="True" w7383 {
                                frame False {
                                }
                                frame True {
                                n6915 = local write "Valve V1 Open"(FALSE ("Valve V1 Open")) -> ()
                                n6916 = local write "Valve V2 Open"(FALSE ("Valve V2 Open")) -> ()
                                n6917 = local write "Valve V3 Open"(FALSE ("Valve V3 Open")) -> ()
                                n6918 = local write "Valve V4 Open"(FALSE ("Valve V4 Open")) -> ()
                                n6919 = local write "Valve V5 Open"(FALSE ("Valve V5 Open")) -> ()
                                n6920 = local write "Valve V6 Open"(FALSE ("Valve V6 Open")) -> ()
                                n6921 = local write "Valve V7 Open"(FALSE ("Valve V7 Open")) -> ()
                                }
                                }
                                }
                                }
                                n6922 = local write "Sample Volume Diverted\ninto Column-2"(0.0 ("Sample Volume Diverted\ninto Column-2")) -> ()
                                n6923 = local write "Buffer-C Volume\nleft to be Pumped"(0.0 ("Buffer-C Volume\nleft to be Pumped")) -> ()
                                n6924 = local write "Vol_previous"(0.0 ("Vol_previous")) -> ()
                                n6925 = local write "Vol_now"(0.0 ("Vol_now")) -> ()
                                n6926 = local write "Volume being Injected \nin this process"(0.0 ("Volume being Injected \nin this process")) -> ()
                                n6927 = local write "Elution of Column-2"(FALSE ("Elution of Column-2")) -> ()
                                n6928 = local write "SEC On"(FALSE ("SEC On")) -> ()
                                }
                              }
                            }
                          }
                          n6929 = local read "Stop for End of \nExperiment \nand Data Writing"() -> (w6523:bool)
                        }
                      }
                    }
                  }
                }
              }
              frame True {
                n6930 = local write "Pause Data Collection"(FALSE ("Pause Data Collection")) -> ()
              }
            }
          }
          frame "Inject Buffer A2, Column 1 with 4 SOD Valves" {
            n6931 = local read "Stopper that ends \nthe main loops"() -> (w7392:bool)
            n6932 = case shown="False" w7392 {
              frame False {
                n6933 = local read "Start the Process"() -> (w7393:bool)
                n6934 = case shown="True" w7393 {
                  frame False {
                    n6935 = local read "Stopper that ends \nthe main loops"() -> (w7395:bool)
                    n6936 = local read "Start the Process"() -> (w7394:bool)
                    n6937 = Or(x=w7395, y=w7394) -> (x .or. y?=w7396:bool)
                    n6938 = case shown="False" w7396 {
                      frame False {
                        n6939 = while {
                          stop <- w7399 stop-if-true
                          n6940 = local read "Stop for End of \nExperiment \nand Data Writing"() -> (w7398:bool)
                          n6941 = local read "Stopper that ends \nthe main loops"() -> (w7401:bool)
                          n6942 = local read "Start the Process"() -> (w7400:bool)
                          n6943 = Wait (ms)(milliseconds to wait=u32 10) -> ()  [unwired: 1 out]
                          n6944 = Or(x=w7401, y=w7400) -> (x .or. y?=w7399:bool)
                          n6945 = local write "Stopper that ends \nthe main loops"(w7398) -> ()
                        }
                        n6946 = One Button Dialog(message="Please Select the Process and Press 'Start the Process' Button") -> ()  [unwired: 1 in, 1 out]
                      }
                      frame True {
                      }
                    }
                  }
                  frame True {
                    n6947 = stacked-sequence {
                      frame #0 {
                        n6948 = local read "Buffer-A2 Volume \nto be Pumped"() -> (w7406:dbl)
                        n6949 = local read "Apparent Volume\nof Syringe"() -> (w7405:dbl)
                        n6950 = Quotient & Remainder(x=w7406, y=w7405) -> (x-y*floor(x/y)=w7403:dbl, floor(x/y)=w7404:dbl)
                        n6951 = for {
                          N: w7404 -> [_]
                          n6952 = stacked-sequence {
                            frame #0 {
                              # "Switch to Port-4"
                              # "Port-4 of pump is connected to Buffer-A"
                              n6953 = local read "VISA Refnum in\nfor Pump"() -> (w7408:refnum<visa-resource-name>)
                              n6954 = local read "Port for \nA2-Wash"() -> (w7407:string)
                              n6955 = call "PortChanger (SubVI).vi"("Port Number"=w7407, "VISA Refnum in"=w7408) -> ()  [unwired: 10 in]
                            }
                            frame #1 {
                              n6956 = local read "VISA Refnum in\nfor Pump"() -> (w7409:refnum<visa-resource-name>)
                              n6957 = call "ProcessCompletionWaiter (SubVI).vi"("VISA Refnum in"=w7409) -> ()  [unwired: 11 in]
                            }
                            frame #2 {
                              n6958 = local read "Buffer-A2 PickUp \nFlow Rate (ul/min)"() -> (w7412:dbl)
                              n6959 = local read "Buffer-A2 Pumping\nResolution"() -> (w7411:T2)
                              n6960 = local read "VISA Refnum in\nfor Pump"() -> (w7414:refnum<visa-resource-name>)
                              n6961 = local read "Apparent Volume\nof Syringe"() -> (w7410:dbl)
                              n6962 = local read "Volume of Syringe"() -> (w7413:dbl)
                              n6963 = call "RPickUp(SubVI).vi"("Volume to be picked up"=w7410, "Volume of Syringe"=w7413, "Resolution of PickUP"=w7411, "PickUp Flow Rate (ul/min)"=w7412, "VISA Refnum in"=w7414) -> ()  [unwired: 6 in, 1 out]
                            }
                            frame #3 {
                              n6964 = local read "Stopper that ends \nthe main loops"() -> (w7415:bool)
                              n6965 = local read "VISA Refnum in\nfor Pump"() -> (w7416:refnum<visa-resource-name>)
                              n6966 = case shown="True" w7415 {
                                frame False {
                                }
                                frame True {
                                n6967 = local read "VISA Refnum in\nfor Pump"() -> (w7417:refnum<visa-resource-name>)
                                n6968 = call "HardStopCurrentProcess (SubVI).vi"("VISA Refnum in"=w7417) -> ()  [unwired: 11 in]
                                }
                              }
                              n6969 = call "ProcessCompletionWaiter (SubVI).vi"("VISA Refnum in"=w7416) -> ()  [unwired: 11 in]
                            }
                            frame #4 {
                              # "Reads the initial Plunger Position for computing the volume dispensed"
                              n6970 = local read "VISA Refnum in\nfor Pump"() -> (w7419:refnum<visa-resource-name>)
                              n6971 = call "AbsolutePlungerPosition (SubVI).vi"("VISA Refnum in"=w7419) -> ("Plunger Position"=w7418:i32)  [unwired: 10 in]
                              n6972 = local write "Initial Plunger Position"(w7418) -> ()
                            }
                            frame #5 {
                              # "Switch to Port-2"
                              # "Port-2 of the pump is conncted to column-1 of chip"
                              n6973 = local read "VISA Refnum in\nfor Pump"() -> (w7421:refnum<visa-resource-name>)
                              n6974 = call "PortChanger (SubVI).vi"("Port Number"="2", "VISA Refnum in"=w7421) -> ()  [unwired: 10 in]
                            }
                            frame #6 {
                              n6975 = local read "Stopper that ends \nthe main loops"() -> (w7422:bool)
                              n6976 = local read "VISA Refnum in\nfor Pump"() -> (w7423:refnum<visa-resource-name>)
                              n6977 = case shown="True" w7422 {
                                frame False {
                                }
                                frame True {
                                n6978 = local read "VISA Refnum in\nfor Pump"() -> (w7424:refnum<visa-resource-name>)
                                n6979 = call "HardStopCurrentProcess (SubVI).vi"("VISA Refnum in"=w7424) -> ()  [unwired: 11 in]
                                }
                              }
                              n6980 = call "ProcessCompletionWaiter (SubVI).vi"("VISA Refnum in"=w7423) -> ()  [unwired: 11 in]
                            }
                            frame #7 {
                              # "Keeps the AMF valve after column-1 open and valve after column-2 closed"
                              n6981 = local read "Buffer-A2 Dispense\nFlow Rate (ul/min)"() -> (w7437:dbl)
                              n6982 = local read "Buffer-A2 Pumping\nResolution"() -> (w7436:T2)
                              n6983 = local read "VISA Refnum in\nfor Pump"() -> (w7439:refnum<visa-resource-name>)
                              n6984 = local write "Pause Data Collection"(FALSE ("Pause Data Collection")) -> ()
                              n6985 = local write "Valve V3 Open"(FALSE ("Valve V3 Open")) -> ()
                              n6986 = local write "Valve V4 Open"(FALSE ("Valve V4 Open")) -> ()
                              n6987 = local write "Valve V1 Open"(TRUE ("Valve V1 Open")) -> ()
                              n6988 = local write "Valve V2 Open"(TRUE ("Valve V2 Open")) -> ()
                              n6989 = local read "Volume of Syringe"() -> (w7438:dbl)
                              n6990 = call "GoToAbsolutePosition(SubVI).vi"("Absolute Volume Position in Syringe (in ul)"=0.0 ("Volume to be Dispensed"), "Volume of Syringe"=w7438, "Resolution of Pumping"=w7436, "Flow Rate (ul/min)"=w7437, "VISA Refnum in"=w7439) -> ()  [unwired: 6 in, 1 out]
                              n6991 = local write "External Valve \nOpen"(TRUE ("External Valve \nOpen")) -> ()
                              n6992 = local write "Valve V8 Open"(FALSE ("Valve V8 Open")) -> ()
                              n6993 = local write "Valve V5 Open"(FALSE ("Valve V5 Open")) -> ()
                              n6994 = local write "Valve V6 Open"(FALSE ("Valve V6 Open")) -> ()
                              n6995 = local write "Valve V7 Open"(FALSE ("Valve V7 Open")) -> ()
                            }
                            frame #8 {
                              n6996 = local read "Initial Plunger Position"() -> (w7442:dbl)
                              n6997 = local read "Buffer-A2 Pumping\nResolution"() -> (w7441:T2)
                              n6998 = local read "VISA Refnum in\nfor Pump"() -> (w7443:refnum<visa-resource-name>)
                              n6999 = local read "Volume of Syringe"() -> (w7440:dbl)
                              n7000 = while {
                                tunnel: w7442 -> [w7449]
                                tunnel: w7443 -> [w7448]
                                tunnel: w7441 -> [w7447]
                                tunnel: w7440 -> [w7446]
                                stop <- w7444 stop-if-true
                                n7001 = Wait (ms)(milliseconds to wait=u32 100) -> ()  [unwired: 1 out]
                                n7002 = stacked-sequence {
                                tunnel: w7449 -> [w7455 _]
                                tunnel: w7448 -> [w7454 w7475]
                                tunnel: w7447 -> [w7453 _]
                                tunnel: w7446 -> [w7452 _]
                                tunnel: [_ w7472] -> w7444
                                frame #0 {
                                n7003 = call "AbsolutePlungerPosition (SubVI).vi"("VISA Refnum in"=w7454) -> ("Plunger Position"=w7451:i32)  [unwired: 10 in]
                                n7004 = case shown="\"Standard Pumping\", Default" w7453 {
                                tunnel: w7455 -> [w7460 w7469]
                                tunnel: w7451 -> [w7461 w7468]
                                tunnel: [w7459 w7466] -> w7450
                                tunnel: w7452 -> [w7458 w7467]
                                frame "Standard Pumping", Default {
                                n7005 = Subtract(x=w7460, y=w7461) -> (x-y=w7457:dbl)
                                n7006 = Absolute Value(x=w7457) -> (abs(x)=w7456:dbl)
                                n7007 = Multiply(x=w7456, y=w7458) -> (x*y=w7463:dbl)
                                n7008 = Divide(x=w7463, y=3000.0) -> (x/y=w7459:dbl)
                                }
                                frame "High Resolution Pumping" {
                                n7009 = Subtract(x=w7469, y=w7468) -> (x-y=w7465:dbl)
                                n7010 = Absolute Value(x=w7465) -> (abs(x)=w7464:dbl)
                                n7011 = Multiply(x=w7464, y=w7467) -> (x*y=w7471:dbl)
                                n7012 = Divide(x=w7471, y=24000.0) -> (x/y=w7466:dbl)
                                }
                                }
                                n7013 = local write "Volume being Injected \nin this process"(w7450) -> ()
                                }
                                frame #1 {
                                n7014 = local read "Stop for End of \nExperiment \nand Data Writing"() -> (w7474:bool)
                                n7015 = call "LSPOneStatus (SubVI).vi"("VISA Refnum in"=w7475) -> ("read buffer"=w7477:string)  [unwired: 10 in]
                                n7016 = call <vilib>:"Trim Whitespace.vi"("string"=w7477) -> ("trimmed string"=w7476:string)  [unwired: 1 in]
                                n7017 = Equal?(x=w7476, y="/0`\u0003") -> (x = y?=w7473:bool)
                                n7018 = Or(x=w7473, y=w7474) -> (x .or. y?=w7472:bool)
                                }
                                }
                              }
                            }
                            frame #9 {
                              n7019 = local read "Stop for End of \nExperiment \nand Data Writing"() -> (w7479:bool)
                              n7020 = local write "Pause Data Collection"(TRUE ("Pause Data Collection")) -> ()
                              n7021 = local write "Valve V3 Open"(FALSE ("Valve V3 Open")) -> ()
                              n7022 = local write "Valve V2 Open"(FALSE ("Valve V2 Open")) -> ()
                              n7023 = local write "Valve V4 Open"(FALSE ("Valve V4 Open")) -> ()
                              n7024 = local write "Valve V1 Open"(FALSE ("Valve V1 Open")) -> ()
                              n7025 = Wait (ms)(milliseconds to wait=u32 500) -> ()  [unwired: 1 out]
                              n7026 = case shown="True" w7479 {
                                frame False {
                                }
                                frame True {
                                n7027 = local read "VISA Refnum in\nfor Pump"() -> (w7489:refnum<visa-resource-name>)
                                n7028 = call "HardStopCurrentProcess (SubVI).vi"("VISA Refnum in"=w7489) -> ()  [unwired: 11 in]
                                }
                              }
                              n7029 = local write "Valve V5 Open"(FALSE ("Valve V5 Open")) -> ()
                              n7030 = local write "Valve V6 Open"(FALSE ("Valve V6 Open")) -> ()
                              n7031 = local write "Valve V7 Open"(FALSE ("Valve V7 Open")) -> ()
                            }
                            frame #10 {
                              n7032 = local write "Volume being Injected \nin this process"(0.0 ("Volume being Injected \nin this process")) -> ()
                            }
                          }
                        }
                        n7033 = local write "Reminder of the \nVolume to be \nPumped"(w7403) -> ()
                      }
                      frame #1 {
                        n7034 = stacked-sequence {
                          frame #0 {
                            # "Switch to Port-4"
                            # "Port-4 of pump is connected to Buffer-A"
                            n7035 = local read "VISA Refnum in\nfor Pump"() -> (w7492:refnum<visa-resource-name>)
                            n7036 = local read "Port for \nA2-Wash"() -> (w7491:string)
